vi "待机唤醒实验.vi"   [LabVIEW 2011]
uses:
  <vilib>/STM32_DriverVI_Interface_F4/GPIO/PortX_in_F4.ctl
  <vilib>/STM32_DriverVI_Interface_F4/GPIO/pin_in_F4.ctl
  <vilib>/STM32_DriverVI_Interface_F4/GPIO/GPI_Mode_Interface_F4.ctl
  <vilib>/STM32_DriverVI_Interface_F4/Interrupt/IO Trigger type_F4.ctl
  <vilib>/STM32_DriverVI_Interface_F4/Interrupt/IO Interrupt Channel_F4.ctl
  <vilib>/STM32_DriverVI_Interface_F4/Interrupt/PreemptionPriority_2_F4.ctl
  <vilib>/STM32_DriverVI_Interface_F4/Interrupt/SubPriority_2_F4.ctl
  <vilib>/eio/EIO_TerminalDirection.ctl
  <vilib>/STM32_DriverVI_Interface_F4/Interrupt/IO Priority Set_2_F4.vi
  <vilib>/STM32_DriverVI_Interface_F4/GPIO_EIO/GPI_EIO_Inner_F4.vi
  <vilib>/STM32_DriverVI_Interface_F4/GPIO_EIO/GPO_EIO_Inner_F4.vi
  <vilib>/eio/EIONode/EIONode.xnode
types:
  T1 = typedef "中断使能禁止_F4.ctl" = enum8{"Disable", "Enable"}
  T2 = typedef "SubPriority_2_F4.ctl" = enum8{"Priority_0（High）", "Priority_1", "Priority_2", "Priority_3（Low）"}
  T3 = typedef "PreemptionPriority_2_F4.ctl" = enum8{"Priority_0（Highest）", "Priority_1", "Priority_2", "Priority_3（Lowest）"}
  T4 = typedef "IO Interrupt Channel_F4.ctl" = u8
  T5 = typedef "IO Trigger type_F4.ctl" = enum8{"Any level Trigger", "Falling edge Trigger", "Rising edge Trigger"}
  T6 = typedef "GPI_Mode_Interface_F4.ctl" = enum8{"Floating Input", "Pull-up Input", "Pull-down Input"}
  T7 = typedef "pin_in_F4.ctl" = enum8{"P0", "P1", "P2", "P3", "P4", "P5", "P6", "P7", "P8", "P9", "P10", "P11", "P12", "P13", "P14", "P15"}
  T8 = typedef "PortX_in_F4.ctl" = enum8{"Port_A", "Port_B", "Port_C", "Port_D", "Port_E", "Port_F", "Port_G", "Port_H", "Port_I"}
  T9 = enum8{"P0", "P1", "P2", "P3", "P4", "P5", "P6", "P7", "P8", "P9", "P10", "P11", "P12", "P13", "P14", "P15"}
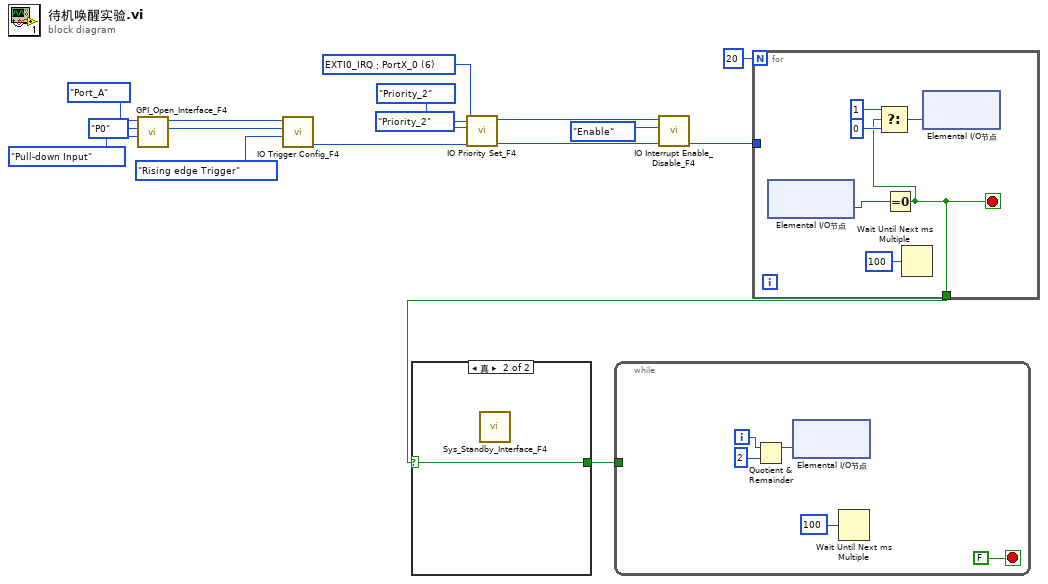
[diagram p0: block diagram]
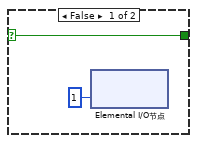
[diagram p2: hidden frame]
diagram:
  w10 = T4 6 items=["EXTI0_IRQ：PortX_0"=6, "EXTI1_IRQ：PortX_1"=7, "EXTI2_IRQ：PortX_2"=8, "EXTI3_IRQ：PortX_3"=9, "EXTI4_IRQ：PortX_4"=10, "EXTI9~5_IRQ：PortX_9~PortX_5"=23, "EXTI15~10_IRQ：PortX_15~PortX_10"=40] ("IO 中断号设置")
  n1 = call <vilib>:"GPI_Open_Interface_F4.vi"("mode"=GPI_Mode_Interface_F4."Pull-down Input", "pin_in"=pin_in_F4."P0", "PortX_in"=PortX_in_F4."Port_A") -> ("pin_out"=w13:u16, "PortX_out"=w14:u16)  [unwired: 6 in, 1 out]
  n2 = call <vilib>:"IO Trigger Config_F4.vi"("Trigger type"=IO_Trigger_type_F4."Rising edge Trigger", "pin_in"=w13, "PortX_in"=w14) -> ("err_out"=w11:u8)  [unwired: 8 in]
  n3 = call-poly <vilib>:"IO Priority Set_F4.vi"("err_in"=w11, "响应优先级"=SubPriority_2_F4."Priority_2", "抢占优先级"=PreemptionPriority_2_F4."Priority_2", "IO 中断号设置"=w10) -> ("err_out"=w7:u8, "中断号"=w6:u16)  [unwired: 6 in]
  n4 = call <vilib>:"IO Interrupt Enable_Disable_F4.vi"("err_in"=w7, "中断使能禁止"=中断使能禁止_F4."Enable", "中断号"=w6) -> ("err_out"=w4:u8)  [unwired: 8 in]
  n5 = for {
    N: 20 -> [_]
    tunnel: w4 -> [_]
    tunnel: [w19] -> w2
    stop <- w19 stop-if-true
    n6 = xnode "Elemental I/O节点"() -> ("KEY_UP"=w18:u8)  [unwired: 1 in, 1 out]
    n7 = Equal To 0?(x=w18) -> (x = 0?=w19:bool)
    n8 = Select(t=u16 1, s=w19, f=u16 0) -> (s? t:f=w20:u16)
    n9 = Wait Until Next ms Multiple(millisecond multiple=u32 100 ("毫秒倍数")) -> ()  [unwired: 1 out]
    n10 = xnode "Elemental I/O节点"("LED_2"=w20) -> ()  [unwired: 1 in, 1 out]
  }
  n11 = case shown="真" w2 {
    selector: w2 -> [w33 w38]
    tunnel: [w33 w38] -> w1
    frame False {
      n12 = xnode "Elemental I/O节点"("LED_2"=u8 1) -> ()  [unwired: 1 in, 1 out]
    }
    frame True {
      n13 = call <vilib>:"Sys_Standby_Interface_F4.vi"() -> ()  [unwired: 11 in, 1 out]
    }
  }
  n14 = while {
    tunnel: w1 -> [_]
    i -> [w42]
    stop <- FALSE stop-if-true
    n15 = Quotient & Remainder(x=w42, y=2) -> (x-y*floor(x/y)=w43:i32)  [unwired: 1 out]
    n16 = xnode "Elemental I/O节点"("LED_1"=w43) -> ()  [unwired: 1 in, 1 out]
    n17 = Wait Until Next ms Multiple(millisecond multiple=u32 100 ("毫秒倍数")) -> ()  [unwired: 1 out]
  }
